vi "Process.vi"(8 "error in (no error)":errorcluster, 11 "ATS660 Class in":refnum<class "ATS660 Class.lvclass">) -> (0 "error out":errorcluster, 3 "ATS660 Class out":refnum<class "ATS660 Class.lvclass">)   [LabVIEW 2014]
uses:
  ATS660 Class.lvclass
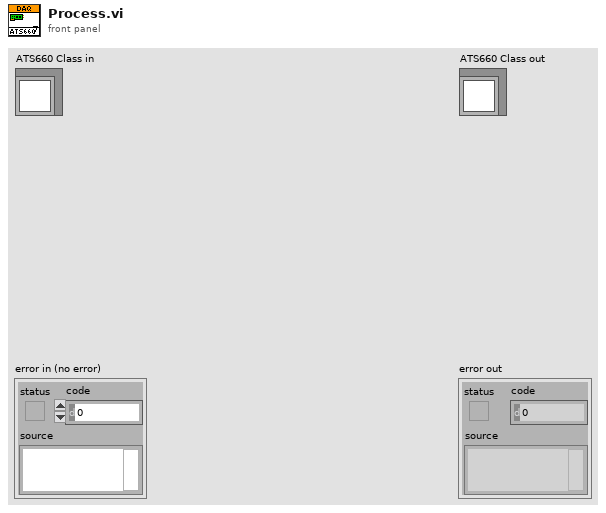
[diagram p1: front panel]
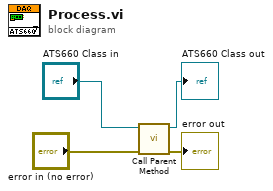
[diagram p0: block diagram]
diagram:
  n1 = call-parent "Call Parent Method"("error in (no error)"="error in (no error)", "DAQ Class in"="ATS660 Class in") -> ("error out"=→"error out":errorcluster, "DAQ Class out"=→"ATS660 Class out":refnum<class "ATS660 Class.lvclass">)  [unwired: 8 in]
